vi "Scripting_G1NewToG3New.vi"(0 "VI Refnum":refnum<vi>, 1 "SearchVI":path=path "C:/classes/MainVI/MyGoop2/utils/MyGoop2_New.vi", 2 "GetToModify":path=path "C:/classes/MainVI/MyGoop2/utils/MyGoop2_GetAttributesToModify.vi", 3 "SetToModify":path=path "C:/classes/MainVI/MyGoop2/utils/MyGoop2_SetModifiedAttributes.vi", 5 "error IO":errorcluster) -> (19 "error out":errorcluster)   [LabVIEW 2016]
uses:
  <vilib>/Utility/miscctls.llb/LVPositionTypeDef.ctl
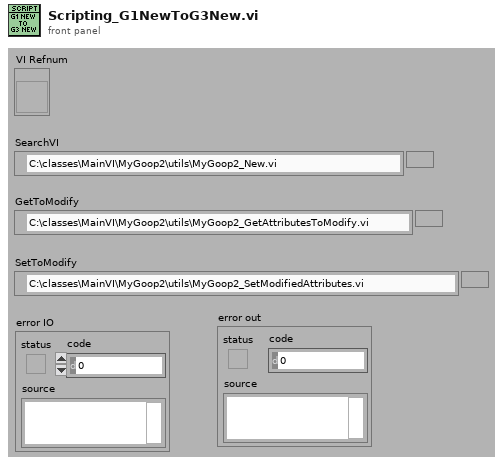
[diagram p1: front panel]
types:
  T1 = cluster{"FoundVI":refnum<vi>, "GetRef":refnum<vi>, "SetRef":refnum<vi>, "Block Diagram":refnum<vi>, "InControl":refnum<vi>, "OutControl":refnum<vi>}
  T2 = typedef "LVPositionTypeDef.ctl" = cluster{"Left":i32, "Top":i32}
  T3 = typedef "LVRectTypeDef.ctl" = cluster{"Left":i16, "Top":i16, "Right":i16, "Bottom":i16}
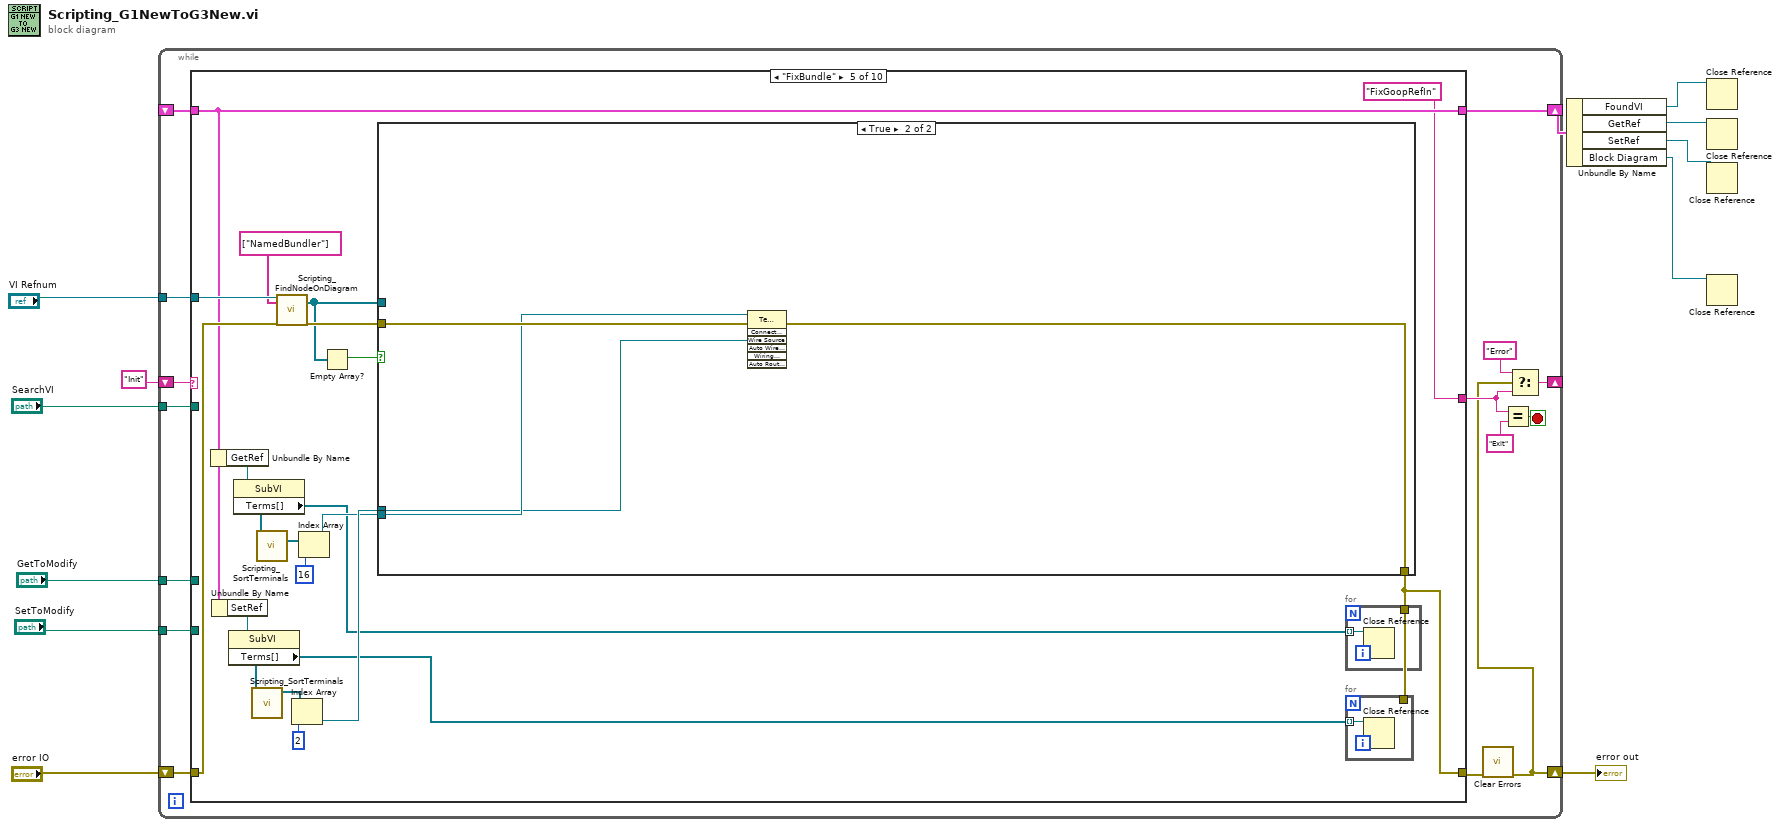
[diagram p0: block diagram]
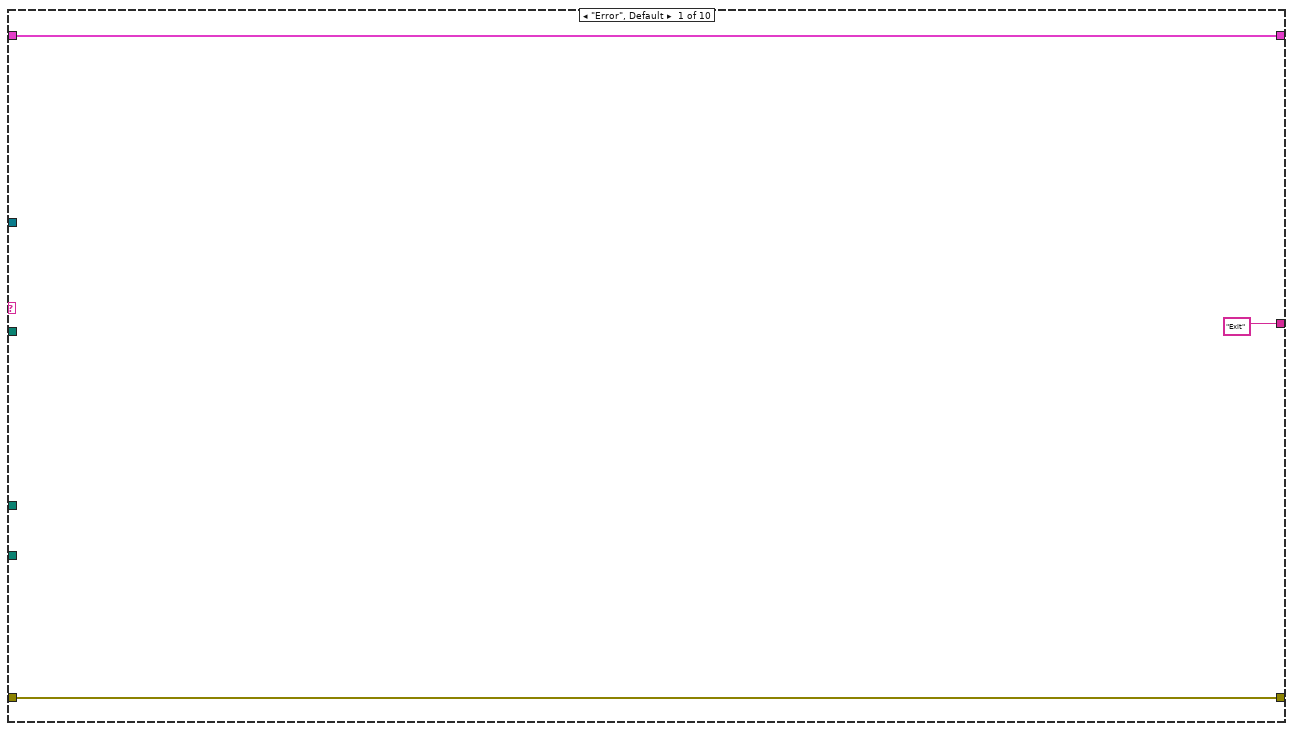
[diagram p2: hidden frame]
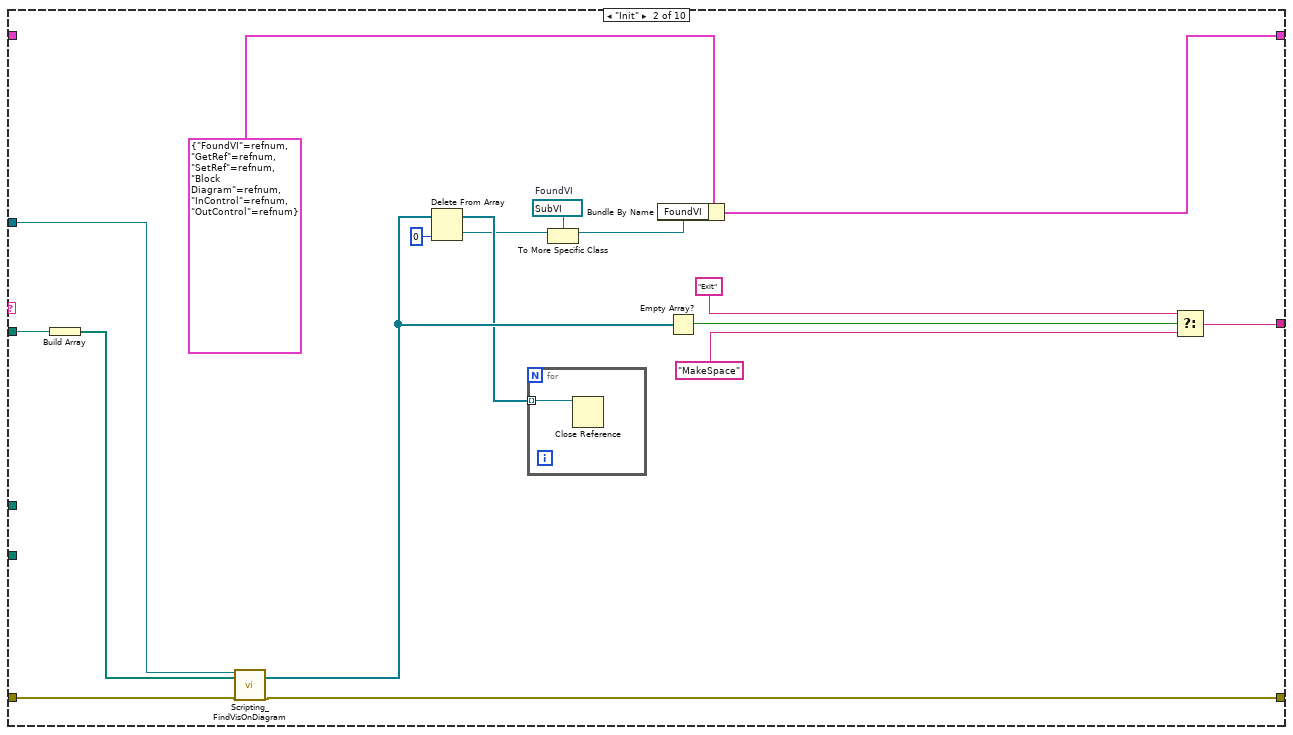
[diagram p3: hidden frame]
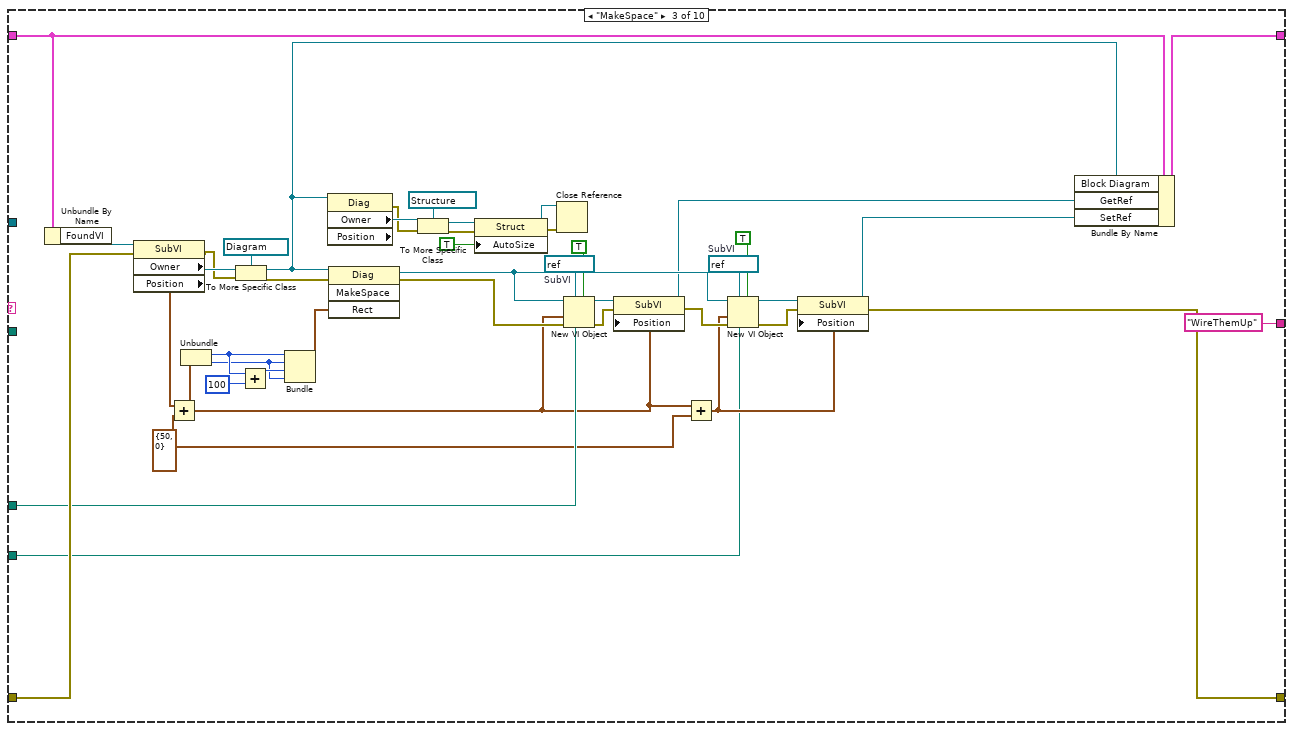
[diagram p4: hidden frame]
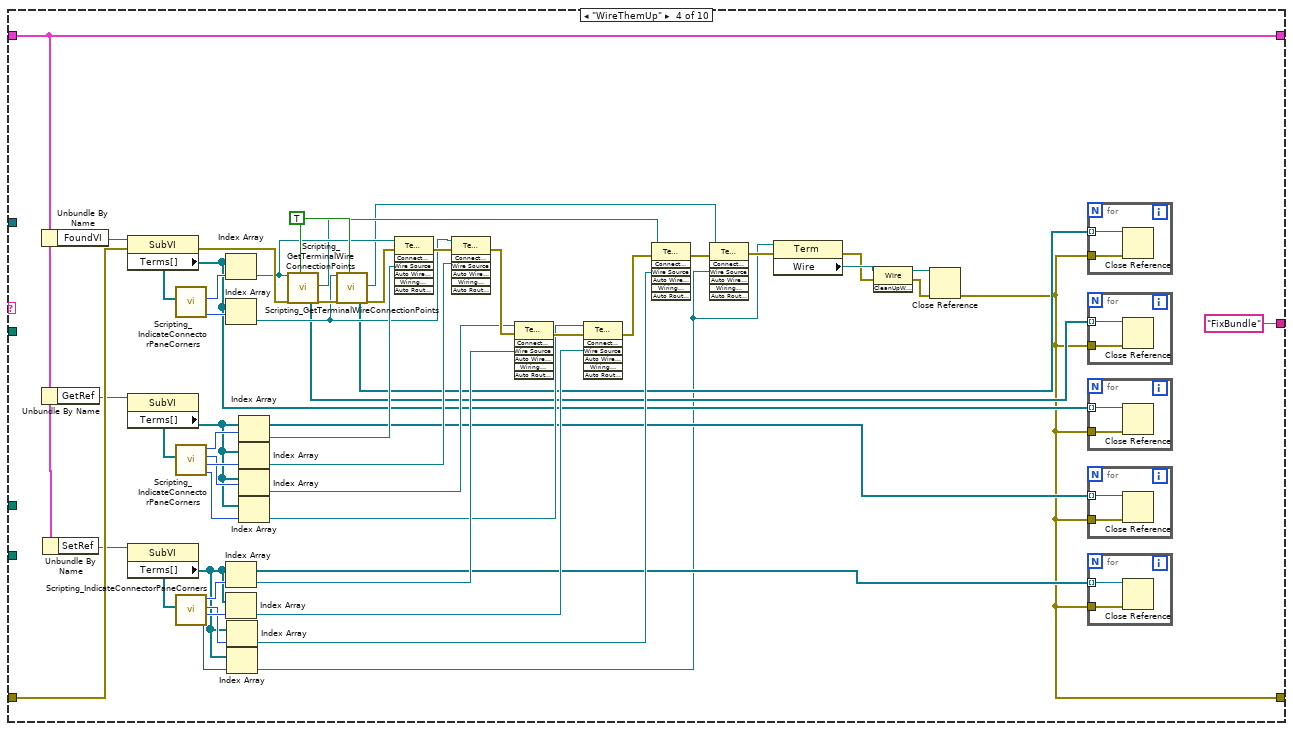
[diagram p5: hidden frame]
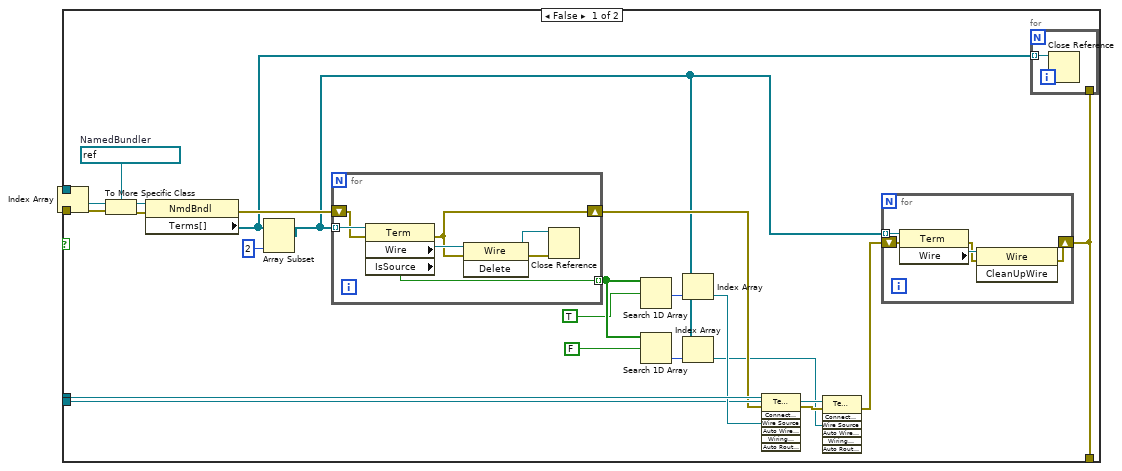
[diagram p6: hidden frame]
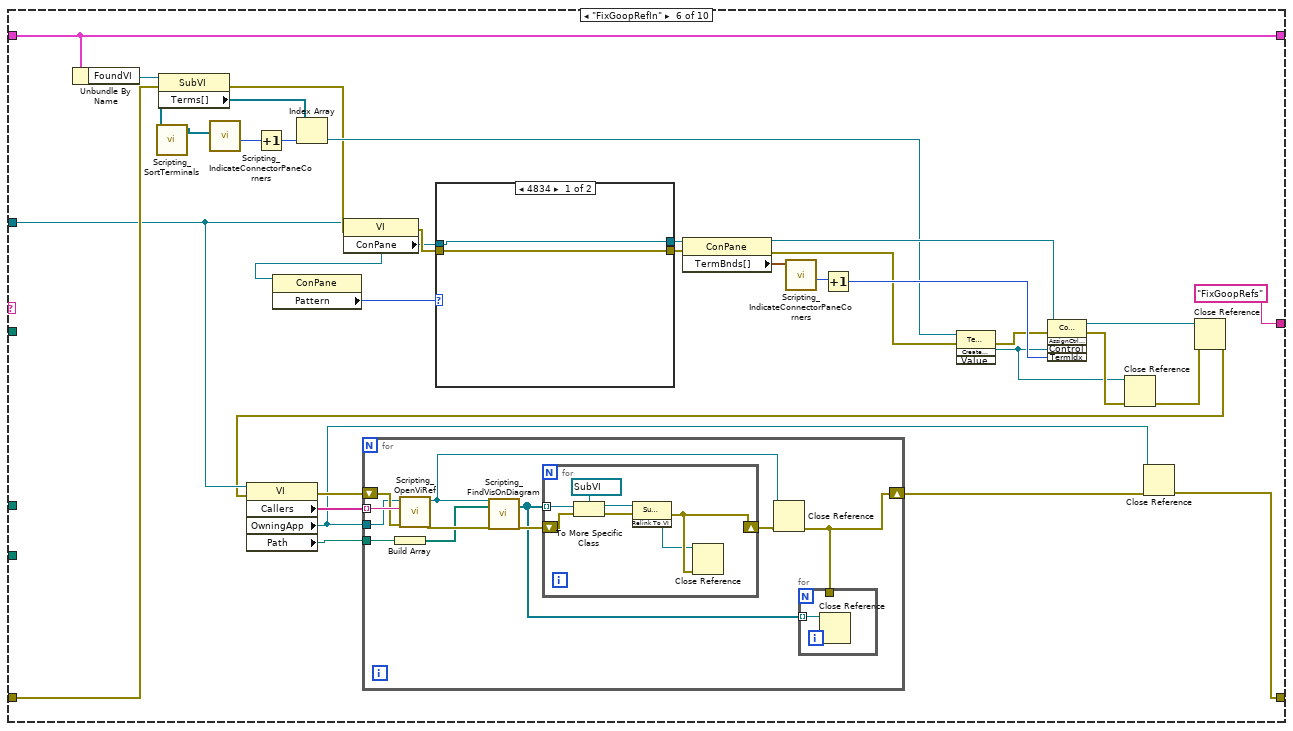
[diagram p7: hidden frame]
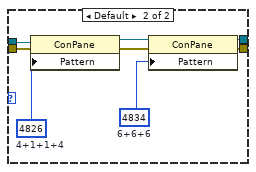
[diagram p8: hidden frame]
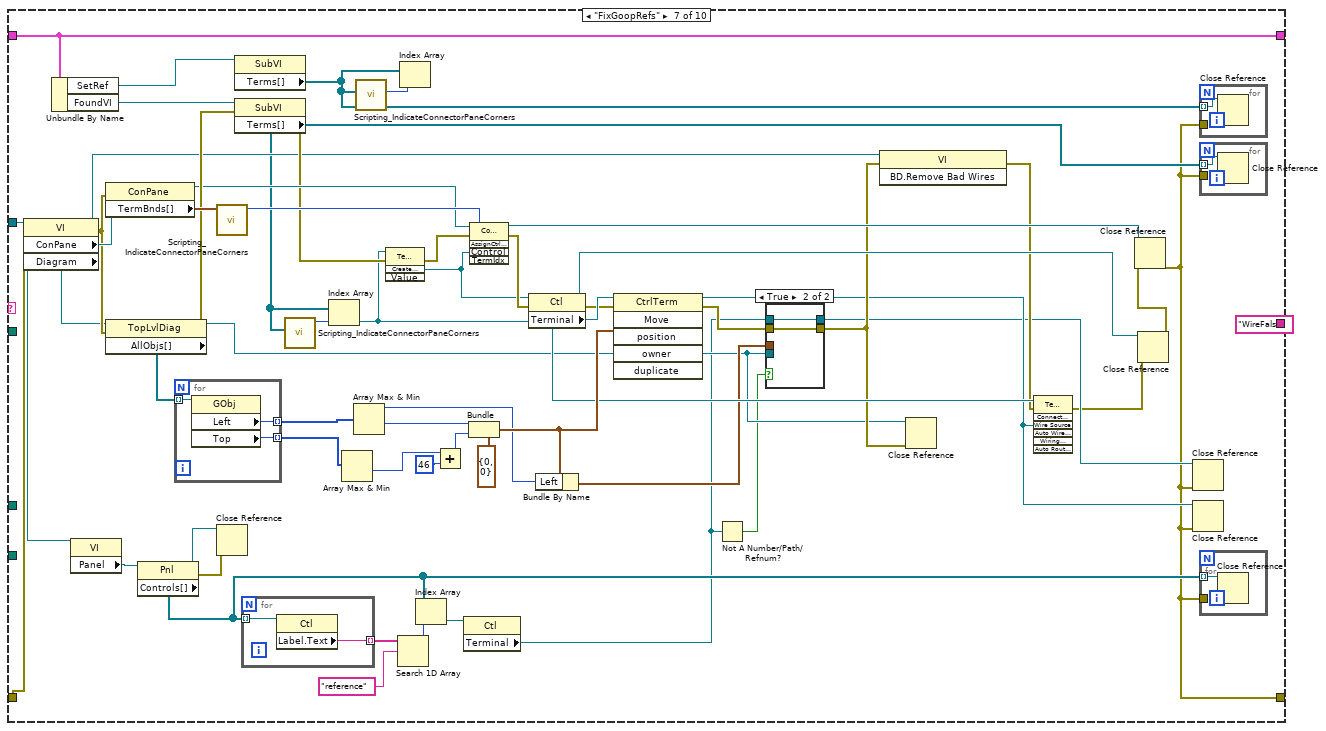
[diagram p9: hidden frame]
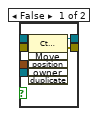
[diagram p10: hidden frame]
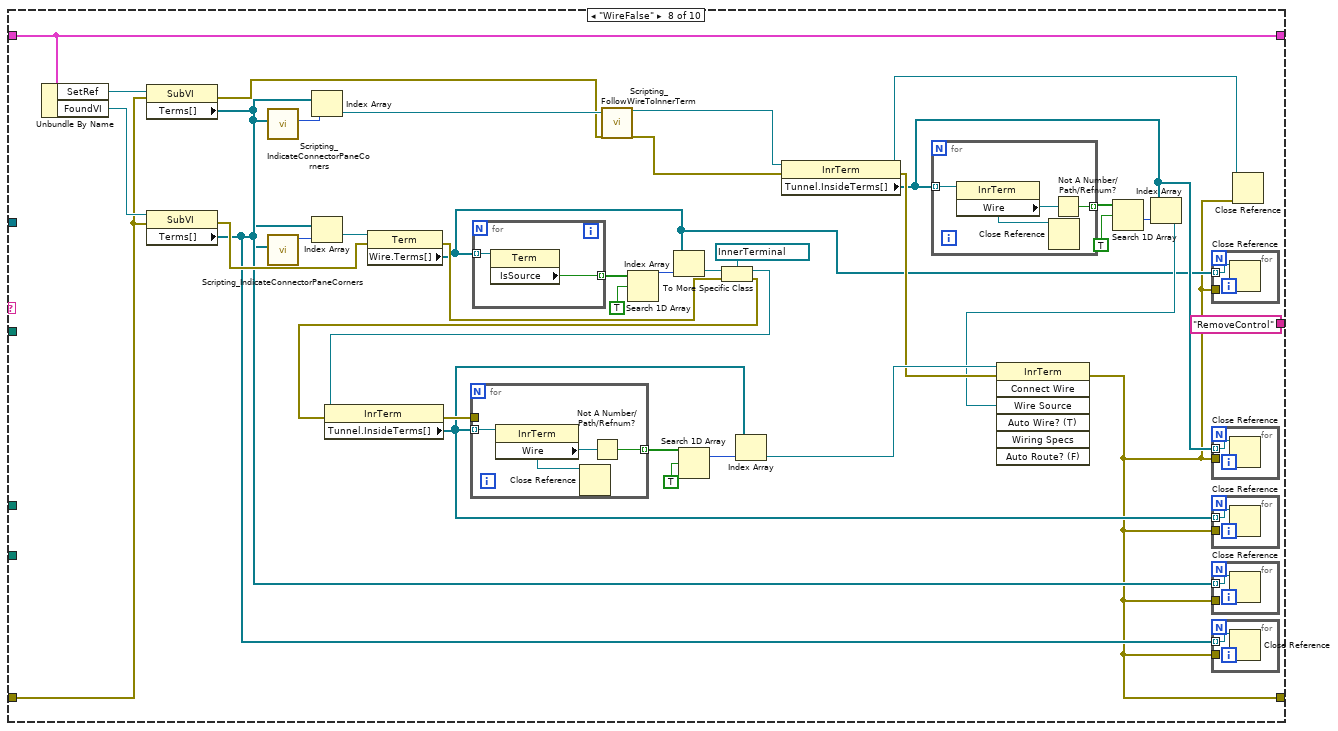
[diagram p11: hidden frame]
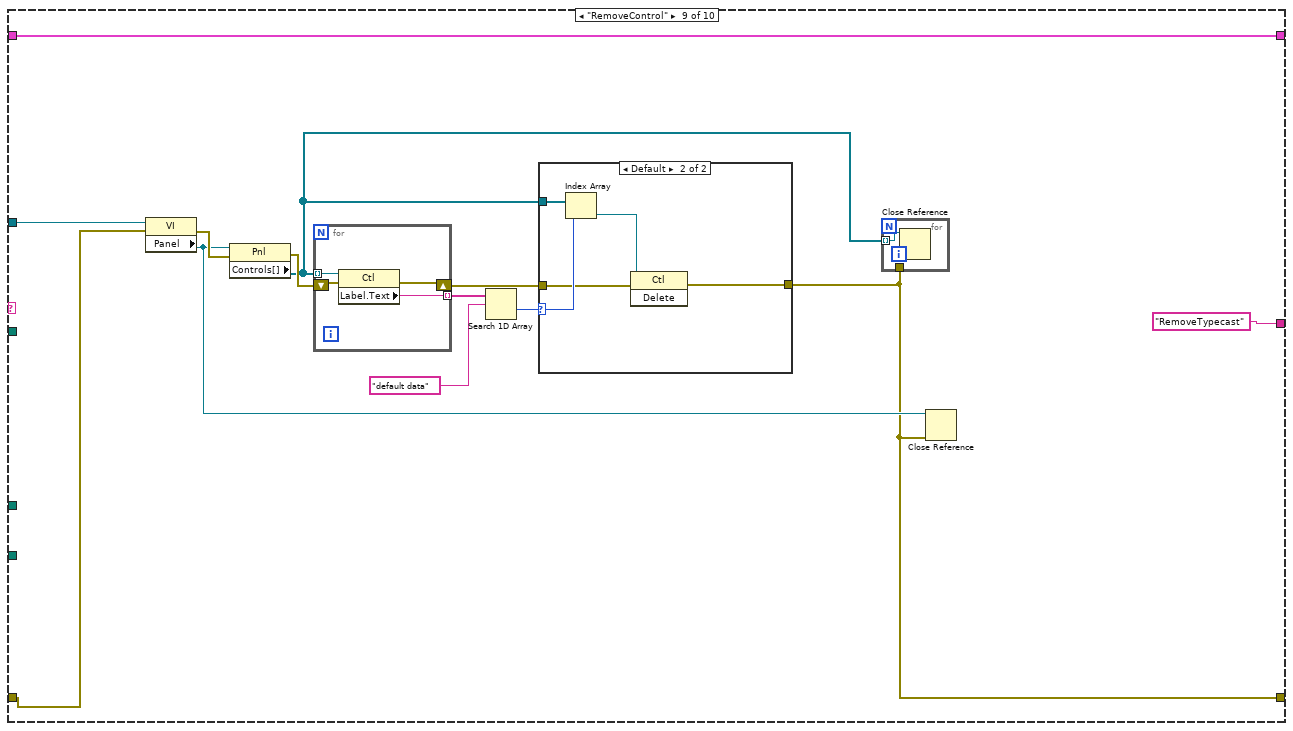
[diagram p12: hidden frame]
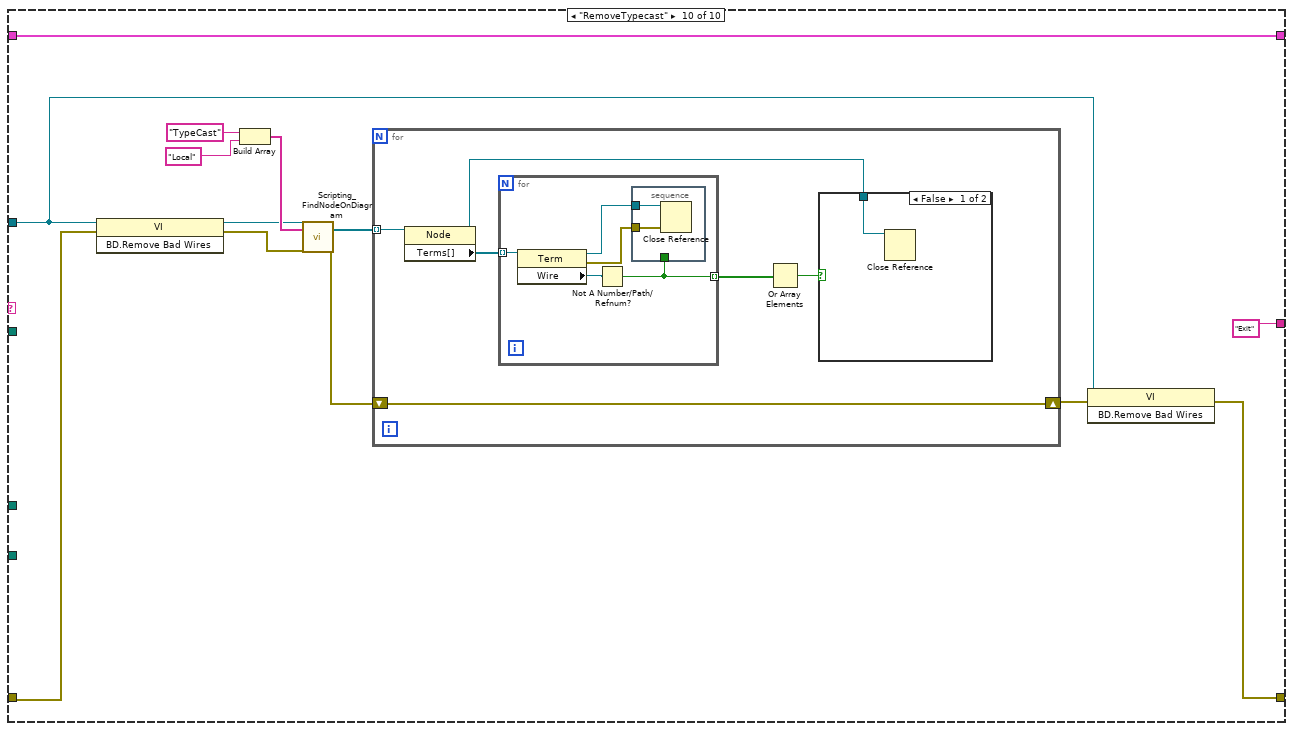
[diagram p14: hidden frame]
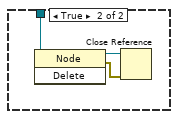
[diagram p15: hidden frame]
diagram:
  n1 = while {
    shift-right: [w13] -> w10
    shift-left: "error IO" -> [w27]
    shift-right: [w25] -> _
    shift-left: "Init" -> [w26]
    shift-right: [w20] -> w6
    shift-left: _ -> [w19]
    tunnel: "VI Refnum" -> [w18]
    tunnel: "SearchVI" -> [w17]
    tunnel: "GetToModify" -> [w16]
    tunnel: "SetToModify" -> [w15]
    stop <- w24 stop-if-true
    n2 = case shown="\"FixBundle\"" w26 {
      tunnel: w27 -> [w28 w45 w90 w138 w166 w226 w319 w357 w401 w429]
      tunnel: [w28 w44 w51 w93 w153 w214 w277 w347 w398 w422] -> w14
      tunnel: ["Exit" w39 "WireThemUp" "FixBundle" "FixGoopRefIn" "FixGoopRefs" "WireFalse" "RemoveControl" "RemoveTypecast" "Exit"] -> w21
      tunnel: [w29 w46 w57 w123 w162 w225 w280 w382 w397 w426] -> w20
      tunnel: w19 -> [w29 _ w58 w123 w162 w225 w280 w382 w397 w426]
      tunnel: w18 -> [_ w43 _ _ w168 w220 w295 _ w402 w424]
      tunnel: w17 -> [_ w36 _ _ _ _ _ _ _ _]
      tunnel: w16 -> [_ _ w83 _ _ _ _ _ _ _]
      tunnel: w15 -> [_ _ w59 _ _ _ _ _ _ _]
      frame "Error", Default {
      }
      frame "Init" {
        w32 = refnum<vi> refnum  # FoundVI
        n3 = Build Array(w36) -> (w35:path[])
        n4 = call <resource>:"Scripting_FindVisOnDiagram.vi"("ViRef"=w43, "VIsToSerachFor/ViName"=w35, "error in (no error)"=w45) -> ("VisFound"=w38:refnum<vi>[], "error out"=w44:errorcluster)  [unwired: 15 in]
        n5 = Delete From Array(array=w38, index=0) -> (deleted portion=w33:refnum<vi>, array with subset deleted=w34:refnum<vi>[])  [unwired: 1 in]
        n6 = for {
          tunnel: w34 -> [w48] mode=indexing
          n7 = Close Reference(reference=w48) -> ()  [unwired: 1 in, 1 out]
        }
        n8 = To More Specific Class(target class=w32, reference=w33) -> (specific class reference=w31:refnum<vi>)  [unwired: 1 in, 1 out]
        n9 = Bundle By Name(cluster=T1 {"FoundVI"=refnum, "GetRef"=refnum, "SetRef"=refnum, "Block Diagram"=refnum, "InControl"=refnum, "OutControl"=refnum}, "FoundVI"=w31) -> (w46:T1)
        n10 = Empty Array?(array=w38) -> (empty?=w42:bool)
        n11 = Select(t="Exit", s=w42, f="MakeSpace") -> (s? t:f=w39:string)
      }
      frame "MakeSpace" {
        w61 = T2 {"Left"=50, "Top"=0} ("y")
        w65 = refnum<vi> refnum  # SubVI
        w86 = refnum<vi> refnum  # SubVI
        n12 = Unbundle By Name(w58) -> ("FoundVI"=w91:refnum<vi>)
        n13 = property class="SubVI"(reference=w91, error in=w90) -> (error out=w87:errorcluster, "Owner"=w88:refnum<vi>, "Position"=w79:T2)  [unwired: 1 out]
        n14 = Add(x=w79, y=w61) -> (x+y=w62:T2)
        n15 = Unbundle(w62) -> ("Left"=w78:i32, "Top"=w75:i32)
        n16 = To More Specific Class(target class=refnum<vi> refnum ("Block Diagram"), reference=w88, error in=w87) -> (specific class reference=w52:refnum<vi>, error out=w72:errorcluster)
        n17 = Add(x=w78, y=i16 100 ("Right")) -> (x+y=w76:i32)
        n18 = Bundle("Left"=w78, "Top"=w75, w76, "Top"=w75) -> (w74:cluster{"Left":i32, "Top":i32, i32, "Top":i32})  [unwired: 1 in]
        n19 = property class="Diag" props=["Owner", "Position"](reference=w52) -> (error out=w49:errorcluster, "Owner"=w71:refnum<vi>)  [unwired: 1 in, 2 out]
        n20 = invoke class="Diag" method="MakeSpace"(reference=w52, error in=w72, "Rect"=w74) -> (reference out=w63:refnum<vi>, error out=w84:errorcluster)  [unwired: 1 in, 2 out]
        n21 = To More Specific Class(target class=refnum<vi> refnum ("Block Diagram"), reference=w71, error in=w49) -> (specific class reference=w70:refnum<vi>, error out=w50:errorcluster)
        n22 = property class="Struct"(reference=w70, error in=w50, "AutoSize"=TRUE ("AutoSize To Fit Contents?")) -> (reference out=w53:refnum<vi>, error out=w54:errorcluster)
        n23 = Close Reference(reference=w53, error in (no error)=w54) -> ()  [unwired: 1 out]
        n24 = New VI Object(vi object class=w86, auto wire? (F)=TRUE, owner refnum=w63, position/next to=w62, 6:w83, 8:w84) -> (object refnum=w82:refnum<vi>, 0:w81:errorcluster)  [unwired: 2 in]
        n25 = property class="SubVI"(reference=w82, error in=w81, "Position"=w62) -> (reference out=w56:refnum<vi>, error out=w64:errorcluster)
        n26 = Add(x=w62, y=w61) -> (x+y=w60:T2)
        n27 = New VI Object(vi object class=w65, auto wire? (F)=TRUE, owner refnum=w63, position/next to=w60, 6:w59, 8:w64) -> (object refnum=w67:refnum<vi>, 0:w68:errorcluster)  [unwired: 2 in]
        n28 = property class="SubVI"(reference=w67, error in=w68, "Position"=w60) -> (reference out=w55:refnum<vi>, error out=w51:errorcluster)
        n29 = Bundle By Name(cluster=w58, "Block Diagram"=w52, "GetRef"=w56, "SetRef"=w55) -> (w57:T1)
      }
      frame "WireThemUp" {
        w134 = TRUE ("RemoveWire(Ture)")
        n30 = Unbundle By Name(w123) -> ("FoundVI"=w139:refnum<vi>)
        n31 = Unbundle By Name(w123) -> ("GetRef"=w133:refnum<vi>)
        n32 = Unbundle By Name(w123) -> ("SetRef"=w124:refnum<vi>)
        n33 = property class="SubVI"(reference=w139, error in=w138) -> (error out=w137:errorcluster, "Terms[]"=w99:refnum<vi>[])  [unwired: 1 out]
        n34 = property class="SubVI"(reference=w133) -> ("Terms[]"=w103:refnum<vi>[])  [unwired: 1 in, 2 out]
        n35 = property class="SubVI"(reference=w124) -> ("Terms[]"=w102:refnum<vi>[])  [unwired: 1 in, 2 out]
        n36 = call <resource>:"Scripting_IndicateConnectorPaneCorners.vi"("Terminals[]"=w99) -> ("RightLower"=w135:i32, "RightTop"=w100:i32)  [unwired: 7 in, 2 out]
        n37 = call <resource>:"Scripting_IndicateConnectorPaneCorners.vi"("Terminals[]"=w103) -> ("RightLower"=w119:i32, "LeftLower"=w131:i32, "RightTop"=w120:i32, "LeftTop"=w132:i32)  [unwired: 7 in]
        n38 = call <resource>:"Scripting_IndicateConnectorPaneCorners.vi"("Terminals[]"=w102) -> ("RightLower"=w111:i32, "LeftLower"=w126:i32, "RightTop"=w112:i32, "LeftTop"=w125:i32)  [unwired: 7 in]
        n39 = Index Array(array=w99, index=w100) -> (element=w113:refnum<vi>)
        n40 = Index Array(array=w99, index=w135) -> (element=w114:refnum<vi>)
        n41 = Index Array(array=w102, index=w125) -> (element=w117:refnum<vi>)
        n42 = Index Array(array=w102, index=w126) -> (element=w116:refnum<vi>)
        n43 = Index Array(array=w102, index=w112) -> (element=w107:refnum<vi>)
        n44 = Index Array(array=w102, index=w111) -> (element=w97:refnum<vi>)
        n45 = Index Array(array=w103, index=w132) -> (element=w129:refnum<vi>)
        n46 = Index Array(array=w103, index=w131) -> (element=w127:refnum<vi>)
        n47 = Index Array(array=w103, index=w120) -> (element=w118:refnum<vi>)
        n48 = Index Array(array=w103, index=w119) -> (element=w115:refnum<vi>)
        n49 = call <resource>:"Scripting_GetTerminalWireConnectionPoints.vi"("Term Refnum In"=w113, "error in"=w137, "RemoveWire(False)"=w134) -> ("AllWireTerminals"=w104:refnum<vi>[], "FirstWireTermDrain"=w110:refnum<vi>, "error out"=w136:errorcluster)  [unwired: 8 in, 6 out]
        n50 = call <resource>:"Scripting_GetTerminalWireConnectionPoints.vi"("Term Refnum In"=w114, "error in"=w136, "RemoveWire(False)"=w134) -> ("AllWireTerminals"=w105:refnum<vi>[], "FirstWireTermDrain"=w109:refnum<vi>, "error out"=w130:errorcluster)  [unwired: 8 in, 6 out]
        n51 = invoke class="Term" method="Connect Wire"(reference=w113, error in=w130, "Wire Source"=w129) -> (error out=w128:errorcluster)  [unwired: 4 in, 6 out]
        n52 = invoke class="Term" method="Connect Wire"(reference=w114, error in=w128, "Wire Source"=w127) -> (error out=w121:errorcluster)  [unwired: 4 in, 6 out]
        n53 = invoke class="Term" method="Connect Wire"(reference=w118, error in=w121, "Wire Source"=w117) -> (error out=w122:errorcluster)  [unwired: 4 in, 6 out]
        n54 = invoke class="Term" method="Connect Wire"(reference=w115, error in=w122, "Wire Source"=w116) -> (error out=w108:errorcluster)  [unwired: 4 in, 6 out]
        n55 = invoke class="Term" method="Connect Wire"(reference=w110, error in=w108, "Wire Source"=w107) -> (error out=w106:errorcluster)  [unwired: 4 in, 6 out]
        n56 = invoke class="Term" method="Connect Wire"(reference=w109, error in=w106, "Wire Source"=w97) -> (error out=w98:errorcluster)  [unwired: 4 in, 6 out]
        n57 = property class="Term"(reference=w97, error in=w98) -> (error out=w95:errorcluster, "Wire"=w96:refnum<vi>)  [unwired: 1 out]
        n58 = invoke class="Wire" method="CleanUpWire"(reference=w96, error in=w95) -> (reference out=w94:refnum<vi>, error out=w92:errorcluster)  [unwired: 1 in, 1 out]
        n59 = Close Reference(reference=w94, error in (no error)=w92) -> (error out=w93:errorcluster)
        n60 = for {
          tunnel: w93 -> [w149]
          tunnel: w105 -> [w148] mode=indexing
          n61 = Close Reference(reference=w148, error in (no error)=w149) -> ()  [unwired: 1 out]
        }
        n62 = for {
          tunnel: w93 -> [w147]
          tunnel: w104 -> [w146] mode=indexing
          n63 = Close Reference(reference=w146, error in (no error)=w147) -> ()  [unwired: 1 out]
        }
        n64 = for {
          tunnel: w93 -> [w145]
          tunnel: w99 -> [w144] mode=indexing
          n65 = Close Reference(reference=w144, error in (no error)=w145) -> ()  [unwired: 1 out]
        }
        n66 = for {
          tunnel: w93 -> [w143]
          tunnel: w103 -> [w142] mode=indexing
          n67 = Close Reference(reference=w142, error in (no error)=w143) -> ()  [unwired: 1 out]
        }
        n68 = for {
          tunnel: w93 -> [w141]
          tunnel: w102 -> [w140] mode=indexing
          n69 = Close Reference(reference=w140, error in (no error)=w141) -> ()  [unwired: 1 out]
        }
      }
      frame "FixBundle" {
        n70 = Unbundle By Name(w162) -> ("GetRef"=w164:refnum<vi>)
        n71 = Unbundle By Name(w162) -> ("SetRef"=w163:refnum<vi>)
        n72 = property class="SubVI"(reference=w163) -> ("Terms[]"=w154:refnum<vi>[])  [unwired: 1 in, 2 out]
        n73 = property class="SubVI"(reference=w164) -> ("Terms[]"=w155:refnum<vi>[])  [unwired: 1 in, 2 out]
        n74 = call <resource>:"Scripting_SortTerminals.vi"("Terminals[]"=w154) -> ("TerminalsOut[]"=w160:refnum<vi>[])  [unwired: 8 in, 2 out]
        n75 = call <resource>:"Scripting_SortTerminals.vi"("Terminals[]"=w155) -> ("TerminalsOut[]"=w157:refnum<vi>[])  [unwired: 8 in, 2 out]
        n76 = call <resource>:"Scripting_FindNodeOnDiagram.vi"("ViRef(Ignored If Not Wired)"=w168, "NodeTypesToSearchFor"=string[] ["NamedBundler"], "error in (no error)"=w166) -> ("Nodes"=w152:refnum<vi>[], "error out"=w165:errorcluster)  [unwired: 15 in]
        n77 = Index Array(array=w160, index=2) -> (element=w159:refnum<vi>)
        n78 = Index Array(array=w157, index=16) -> (element=w156:refnum<vi>)
        n79 = Empty Array?(array=w152) -> (empty?=w150:bool)
        n80 = case shown="True" w150 {
          tunnel: w165 -> [w186 w208]
          tunnel: w159 -> [w181 w206]
          tunnel: w156 -> [w177 w207]
          tunnel: [w170 w205] -> w153
          tunnel: w152 -> [w169 _]
          frame False {
            w190 = refnum<vi> refnum  # NamedBundler
            n81 = Index Array(array=w169) -> (element=w191:refnum<vi>)  [unwired: 1 in]
            n82 = To More Specific Class(target class=w190, reference=w191, error in=w186) -> (specific class reference=w189:refnum<vi>, error out=w187:errorcluster)
            n83 = property class="NmdBndl"(reference=w189, error in=w187) -> (error out=w188:errorcluster, "Terms[]"=w175:refnum<vi>[])  [unwired: 1 out]
            n84 = Array Subset(array=w175, length=2) -> (w172:refnum<vi>[])  [unwired: 1 in]
            n85 = for {
              tunnel: w172 -> [w204] mode=indexing
              shift-right: [w198] -> w176
              shift-left: w188 -> [w201]
              tunnel: [w199] -> w184 mode=indexing
              n86 = property class="Term"(reference=w204, error in=w201) -> (error out=w198:errorcluster, "Wire"=w203:refnum<vi>, "IsSource"=w199:bool)  [unwired: 1 out]
              n87 = invoke class="Wire" method="Delete"(reference=w203, error in=w198) -> (reference out=w202:refnum<vi>, error out=w200:errorcluster)  [unwired: 1 in, 1 out]
              n88 = Close Reference(reference=w202, error in (no error)=w200) -> ()  [unwired: 1 out]
            }
            n89 = Search 1D Array(1D array=w184, element=TRUE) -> (index of element=w180:i32)  [unwired: 1 in]
            n90 = Search 1D Array(1D array=w184, element=FALSE) -> (index of element=w174:i32)  [unwired: 1 in]
            n91 = Index Array(array=w172, index=w180) -> (element=w179:refnum<vi>)
            n92 = Index Array(array=w172, index=w174) -> (element=w173:refnum<vi>)
            n93 = invoke class="Term" method="Connect Wire"(reference=w181, error in=w176, "Wire Source"=w179) -> (error out=w178:errorcluster)  [unwired: 4 in, 6 out]
            n94 = invoke class="Term" method="Connect Wire"(reference=w177, error in=w178, "Wire Source"=w173) -> (error out=w171:errorcluster)  [unwired: 4 in, 6 out]
            n95 = for {
              tunnel: w172 -> [w196] mode=indexing
              shift-right: [w192] -> w170
              shift-left: w171 -> [w194]
              n96 = property class="Term"(reference=w196, error in=w194) -> (error out=w193:errorcluster, "Wire"=w195:refnum<vi>)  [unwired: 1 out]
              n97 = invoke class="Wire" method="CleanUpWire"(reference=w195, error in=w193) -> (error out=w192:errorcluster)  [unwired: 1 in, 2 out]
            }
            n98 = for {
              tunnel: w175 -> [w197] mode=indexing
              tunnel: w170 -> [_]
              n99 = Close Reference(reference=w197) -> ()  [unwired: 1 in, 1 out]
            }
          }
          frame True {
            n100 = invoke class="Term" method="Connect Wire"(reference=w207, error in=w208, "Wire Source"=w206) -> (error out=w205:errorcluster)  [unwired: 4 in, 6 out]
          }
        }
        n101 = for {
          tunnel: w155 -> [w210] mode=indexing
          tunnel: w153 -> [_]
          n102 = Close Reference(reference=w210) -> ()  [unwired: 1 in, 1 out]
        }
        n103 = for {
          tunnel: w154 -> [w209] mode=indexing
          tunnel: w153 -> [_]
          n104 = Close Reference(reference=w209) -> ()  [unwired: 1 in, 1 out]
        }
      }
      frame "FixGoopRefIn" {
        n105 = Unbundle By Name(w225) -> ("FoundVI"=w239:refnum<vi>)
        n106 = property class="SubVI"(reference=w239, error in=w226) -> (error out=w227:errorcluster, "Terms[]"=w237:refnum<vi>[])  [unwired: 1 out]
        n107 = call <resource>:"Scripting_SortTerminals.vi"("Terminals[]"=w237) -> ("TerminalsOut[]"=w236:refnum<vi>[])  [unwired: 8 in, 2 out]
        n108 = call <resource>:"Scripting_IndicateConnectorPaneCorners.vi"("Terminals[]"=w236) -> ("LeftLower"=w238:i32)  [unwired: 7 in, 3 out]
        n109 = Increment(x=w238) -> (x+1=w243:i32)
        n110 = Index Array(array=w237, index=w243) -> (element=w229:refnum<vi>)
        n111 = property class="VI"(reference=w220, error in=w227) -> (error out=w223:errorcluster, "ConPane"=w212:refnum<vi>)  [unwired: 1 out]
        n112 = property class="ConPane"(reference=w212) -> ("Pattern"=w211:u32)  [unwired: 1 in, 2 out]
        n113 = case shown="4834" w211 {
          tunnel: w212 -> [w245 w253]
          tunnel: w223 -> [w244 w252]
          tunnel: [w244 w247] -> w222
          tunnel: [w245 w246] -> w221
          frame 4834 {
          }
          frame Default {
            w251 = u32 4826  # 4+1+1+4
            w248 = u32 4834  # 6+6+6
            n114 = property class="ConPane"(reference=w253, error in=w252, "Pattern"=w251) -> (reference out=w250:refnum<vi>, error out=w249:errorcluster)
            n115 = property class="ConPane"(reference=w250, error in=w249, "Pattern"=w248) -> (reference out=w246:refnum<vi>, error out=w247:errorcluster)
          }
        }
        n116 = property class="ConPane"(reference=w221, error in=w222) -> (reference out=w235:refnum<vi>, error out=w228:errorcluster, "TermBnds[]"=w241:T3[])
        n117 = call <resource>:"Scripting_IndicateConnectorPaneCorners.vi"("TermBnds[]"=w241) -> ("LeftLower"=w240:i32)  [unwired: 7 in, 3 out]
        n118 = Increment(x=w240) -> (x+1=w234:i32)
        n119 = invoke class="Term" method="Create Control"(reference=w229, error in=w228) -> (error out=w233:errorcluster, "Create Control"=w232:refnum<vi>)  [unwired: 2 in, 2 out]
        n120 = invoke class="ConPane" method="AssignCtrlToTerm"(reference=w235, error in=w233, "Control"=w232, "TermIdx"=w234) -> (reference out=w230:refnum<vi>, error out=w242:errorcluster)  [unwired: 1 in, 3 out]
        n121 = Close Reference(reference=w232, error in (no error)=w242) -> (error out=w231:errorcluster)
        n122 = Close Reference(reference=w230, error in (no error)=w231) -> (error out=w216:errorcluster)
        n123 = property class="VI"(reference=w220, error in=w216) -> (error out=w218:errorcluster, "Callers"=w219:string[], "OwningApp"=w213:refnum<vi>, "Path"=w217:path)  [unwired: 1 out]
        n124 = for {
          tunnel: w219 -> [w264] mode=indexing
          tunnel: w217 -> [w261]
          tunnel: w213 -> [w257]
          shift-right: [w254] -> w215
          shift-left: w218 -> [w263]
          n125 = Build Array(w261) -> (w260:path[])
          n126 = call <resource>:"Scripting_OpenViRef.vi"("error in"=w263, "ViPath/ViName/Viref"=w264, "AppRef"=w257) -> ("error out"=w262:errorcluster, "vi reference"=w255:refnum<vi>)  [unwired: 6 in, 1 out]
          n127 = call <resource>:"Scripting_FindVisOnDiagram.vi"("ViRef"=w255, "VIsToSerachFor/ViName"=w260, "error in (no error)"=w262) -> ("VisFound"=w258:refnum<vi>[], "error out"=w259:errorcluster)  [unwired: 15 in]
          n128 = for {
            tunnel: w258 -> [w271] mode=indexing
            shift-right: [w267] -> w256
            shift-left: w259 -> [w270]
            n129 = To More Specific Class(target class=refnum<vi> refnum ("WhileLoop"), reference=w271, error in=w270) -> (specific class reference=w269:refnum<vi>, error out=w268:errorcluster)
            n130 = invoke class="SubVI" method="Relink To VI"(reference=w269, error in=w268) -> (error out=w267:errorcluster, "Relink To VI"=w266:refnum<vi>)  [unwired: 1 in, 1 out]
            n131 = Close Reference(reference=w266, error in (no error)=w267) -> ()  [unwired: 1 out]
          }
          n132 = Close Reference(reference=w255, error in (no error)=w256) -> (error out=w254:errorcluster)
          n133 = for {
            tunnel: w258 -> [w265] mode=indexing
            tunnel: w254 -> [_]
            n134 = Close Reference(reference=w265) -> ()  [unwired: 1 in, 1 out]
          }
        }
        n135 = Close Reference(reference=w213, error in (no error)=w215) -> (error out=w214:errorcluster)
      }
      frame "FixGoopRefs" {
        n136 = property class="VI"(reference=w295, error in=w319) -> (reference out=w299:refnum<vi>, error out=w304:errorcluster, "ConPane"=w328:refnum<vi>, "Diagram"=w303:refnum<vi>)
        n137 = Unbundle By Name(w280) -> ("SetRef"=w289:refnum<vi>, "FoundVI"=w309:refnum<vi>)
        n138 = property class="VI"(reference=w295) -> ("Panel"=w294:refnum<vi>)  [unwired: 1 in, 2 out]
        n139 = property class="ConPane"(reference=w328, error in=w304) -> (reference out=w318:refnum<vi>, "TermBnds[]"=w327:T3[])  [unwired: 1 out]
        n140 = property class="TopLvlDiag"(reference=w303, error in=w304) -> (reference out=w283:refnum<vi>, error out=w323:errorcluster, "AllObjs[]"=w314:refnum<vi>[])
        n141 = property class="Pnl"(reference=w294) -> (reference out=w285:refnum<vi>, error out=w286:errorcluster, "Controls[]"=w287:refnum<vi>[])  [unwired: 1 in]
        n142 = for {
          tunnel: w314 -> [w345] mode=indexing
          tunnel: [w344] -> w326 mode=indexing
          tunnel: [w343] -> w325 mode=indexing
          n143 = property class="GObj"(reference=w345) -> ("Left"=w344:i32, "Top"=w343:i32)  [unwired: 1 in, 2 out]
        }
        n144 = call <resource>:"Scripting_IndicateConnectorPaneCorners.vi"("TermBnds[]"=w327) -> ("LeftTop"=w321:i32)  [unwired: 7 in, 3 out]
        n145 = Close Reference(reference=w285, error in (no error)=w286) -> ()  [unwired: 1 out]
        n146 = property class="SubVI"(reference=w289) -> ("Terms[]"=w281:refnum<vi>[])  [unwired: 1 in, 2 out]
        n147 = property class="SubVI"(reference=w309, error in=w323) -> (error out=w310:errorcluster, "Terms[]"=w282:refnum<vi>[])  [unwired: 1 out]
        n148 = for {
          tunnel: [w342] -> w298 mode=indexing
          tunnel: w287 -> [w341] mode=indexing
          n149 = property class="Ctl"(reference=w341) -> ("Label.Text"=w342:string)  [unwired: 1 in, 2 out]
        }
        n150 = call <resource>:"Scripting_IndicateConnectorPaneCorners.vi"("Terminals[]"=w282) -> ("LeftTop"=w329:i32)  [unwired: 7 in, 3 out]
        n151 = Index Array(array=w282, index=w329) -> (element=w301:refnum<vi>)
        n152 = Array Max & Min(array=w325) -> (min value=w306:i32)  [unwired: 3 out]
        n153 = Array Max & Min(array=w326) -> (max value=w290:i32, min value=w307:i32)  [unwired: 2 out]
        n154 = call <resource>:"Scripting_IndicateConnectorPaneCorners.vi"("Terminals[]"=w281) -> ("RightTop"=w288:i32)  [unwired: 7 in, 3 out]
        n155 = invoke class="Term" method="Create Control"(reference=w301, error in=w310) -> (error out=w311:errorcluster, "Create Control"=w312:refnum<vi>)  [unwired: 2 in, 2 out]
        n156 = Search 1D Array(1D array=w298, element="reference") -> (index of element=w297:i32)  [unwired: 1 in]
        n157 = Index Array(array=w281, index=w288) -> ()  [unwired: 1 out]
        n158 = Index Array(array=w287, index=w297) -> (element=w296:refnum<vi>)
        n159 = Add(x=w306, y=u32 46) -> (x+y=w305:u32)
        n160 = property class="Ctl"(reference=w296) -> ("Terminal"=w274:refnum<vi>)  [unwired: 1 in, 2 out]
        n161 = Bundle(cluster=T2 {"Left"=0, "Top"=0} ("position"), "Left"=w307, "Top"=w305) -> (w302:T2)
        n162 = invoke class="ConPane" method="AssignCtrlToTerm"(reference=w318, error in=w311, "Control"=w312, "TermIdx"=w321) -> (reference out=w324:refnum<vi>, error out=w317:errorcluster)  [unwired: 1 in, 3 out]
        n163 = property class="Ctl"(reference=w312, error in=w317) -> (reference out=w315:refnum<vi>, error out=w313:errorcluster, "Terminal"=w316:refnum<vi>)
        n164 = Bundle By Name(cluster=w302, "Left"=w290) -> (w291:T2)
        n165 = invoke class="CtrlTerm" method="Move"(reference=w316, error in=w313, "position"=w302, "owner"=w283) -> (reference out=w279:refnum<vi>, error out=w292:errorcluster)  [unwired: 2 in, 4 out]
        n166 = Not A Number/Path/Refnum?(number/path/refnum=w274) -> (NaN/Path/Refnum?=w273:bool)
        n167 = case shown="True" w273 {
          tunnel: w292 -> [w335 w336]
          tunnel: w291 -> [w334 _]
          tunnel: [w333 w336] -> w284
          tunnel: w283 -> [w332 _]
          tunnel: [w331 w337] -> w278
          tunnel: w274 -> [w330 w337]
          frame False {
            n168 = invoke class="CtrlTerm" method="Move"(reference=w330, error in=w335, "position"=w334, "owner"=w332) -> (reference out=w331:refnum<vi>, error out=w333:errorcluster)  [unwired: 2 in, 4 out]
          }
          frame True {
          }
        }
        n169 = invoke class="VI" method="BD.Remove Bad Wires"(reference=w299, error in=w284) -> (error out=w300:errorcluster)  [unwired: 1 in, 2 out]
        n170 = Close Reference(reference=w283, error in (no error)=w284) -> ()  [unwired: 1 out]
        n171 = invoke class="Term" method="Connect Wire"(reference=w301, error in=w300, "Wire Source"=w279) -> (error out=w276:errorcluster)  [unwired: 4 in, 6 out]
        n172 = Close Reference(reference=w315, error in (no error)=w276) -> (error out=w275:errorcluster)
        n173 = Close Reference(reference=w324, error in (no error)=w275) -> (error out=w277:errorcluster)
        n174 = Close Reference(reference=w278, error in (no error)=w277) -> ()  [unwired: 1 out]
        n175 = Close Reference(reference=w279, error in (no error)=w277) -> ()  [unwired: 1 out]
        n176 = for {
          tunnel: w281 -> [w338] mode=indexing
          tunnel: w277 -> [_]
          n177 = Close Reference(reference=w338) -> ()  [unwired: 1 in, 1 out]
        }
        n178 = for {
          tunnel: w282 -> [w339] mode=indexing
          tunnel: w277 -> [_]
          n179 = Close Reference(reference=w339) -> ()  [unwired: 1 in, 1 out]
        }
        n180 = for {
          tunnel: w287 -> [w340] mode=indexing
          tunnel: w277 -> [_]
          n181 = Close Reference(reference=w340) -> ()  [unwired: 1 in, 1 out]
        }
      }
      frame "WireFalse" {
        n182 = Unbundle By Name(w382) -> ("SetRef"=w380:refnum<vi>, "FoundVI"=w371:refnum<vi>)
        n183 = property class="SubVI"(reference=w380, error in=w357) -> (error out=w349:errorcluster, "Terms[]"=w352:refnum<vi>[])  [unwired: 1 out]
        n184 = property class="SubVI"(reference=w371, error in=w357) -> (error out=w360:errorcluster, "Terms[]"=w351:refnum<vi>[])  [unwired: 1 out]
        n185 = call <resource>:"Scripting_IndicateConnectorPaneCorners.vi"("Terminals[]"=w352) -> ("RightTop"=w381:i32)  [unwired: 7 in, 3 out]
        n186 = call <resource>:"Scripting_IndicateConnectorPaneCorners.vi"("Terminals[]"=w351) -> ("LeftTop"=w370:i32)  [unwired: 7 in, 3 out]
        n187 = Index Array(array=w352, index=w381) -> (element=w379:refnum<vi>)
        n188 = Index Array(array=w351, index=w370) -> (element=w374:refnum<vi>)
        n189 = property class="Term"(reference=w374, error in=w360) -> (error out=w359:errorcluster, "Wire.Terms[]"=w353:refnum<vi>[])  [unwired: 1 out]
        n190 = for {
          tunnel: w353 -> [w393] mode=indexing
          tunnel: [w392] -> w373 mode=indexing
          n191 = property class="Term"(reference=w393) -> ("IsSource"=w392:bool)  [unwired: 1 in, 2 out]
        }
        n192 = call <resource>:"Scripting_FollowWireToInnerTerm.vi"("Term Refnum"=w379, "error in"=w349) -> ("reference"=w378:refnum<vi>, "error out"=w348:errorcluster)  [unwired: 16 in]
        n193 = Search 1D Array(1D array=w373, element=TRUE) -> (index of element=w369:i32)  [unwired: 1 in]
        n194 = Index Array(array=w353, index=w369) -> (element=w367:refnum<vi>)
        n195 = To More Specific Class(target class=refnum<vi> refnum ("reference"), reference=w367, error in=w359) -> (specific class reference=w366:refnum<vi>, error out=w350:errorcluster)
        n196 = property class="InrTerm"(reference=w366, error in=w350) -> (error out=w361:errorcluster, "Tunnel.InsideTerms[]"=w355:refnum<vi>[])  [unwired: 1 out]
        n197 = for {
          tunnel: w355 -> [w391] mode=indexing
          tunnel: [w390] -> w363 mode=indexing
          tunnel: w361 -> [_]
          n198 = property class="InrTerm"(reference=w391) -> ("Wire"=w389:refnum<vi>)  [unwired: 1 in, 2 out]
          n199 = Close Reference(reference=w389) -> ()  [unwired: 1 in, 1 out]
          n200 = Not A Number/Path/Refnum?(number/path/refnum=w389) -> (NaN/Path/Refnum?=w390:bool)
        }
        n201 = Search 1D Array(1D array=w363, element=TRUE) -> (index of element=w364:i32)  [unwired: 1 in]
        n202 = Index Array(array=w355, index=w364) -> (element=w362:refnum<vi>)
        n203 = property class="InrTerm"(reference=w378, error in=w348) -> (reference out=w346:refnum<vi>, error out=w358:errorcluster, "Tunnel.InsideTerms[]"=w356:refnum<vi>[])
        n204 = for {
          tunnel: w356 -> [w396] mode=indexing
          tunnel: [w395] -> w375 mode=indexing
          n205 = property class="InrTerm"(reference=w396) -> ("Wire"=w394:refnum<vi>)  [unwired: 1 in, 2 out]
          n206 = Close Reference(reference=w394) -> ()  [unwired: 1 in, 1 out]
          n207 = Not A Number/Path/Refnum?(number/path/refnum=w394) -> (NaN/Path/Refnum?=w395:bool)
        }
        n208 = Search 1D Array(1D array=w375, element=TRUE) -> (index of element=w377:i32)  [unwired: 1 in]
        n209 = Index Array(array=w356, index=w377) -> (element=w354:refnum<vi>)
        n210 = invoke class="InrTerm" method="Connect Wire"(reference=w362, error in=w358, "Wire Source"=w354) -> (error out=w347:errorcluster)  [unwired: 4 in, 6 out]
        n211 = for {
          tunnel: w353 -> [w386] mode=indexing
          tunnel: w347 -> [_]
          n212 = Close Reference(reference=w386) -> ()  [unwired: 1 in, 1 out]
        }
        n213 = for {
          tunnel: w356 -> [w388] mode=indexing
          tunnel: w347 -> [_]
          n214 = Close Reference(reference=w388) -> ()  [unwired: 1 in, 1 out]
        }
        n215 = for {
          tunnel: w355 -> [w387] mode=indexing
          tunnel: w347 -> [_]
          n216 = Close Reference(reference=w387) -> ()  [unwired: 1 in, 1 out]
        }
        n217 = for {
          tunnel: w352 -> [w385] mode=indexing
          tunnel: w347 -> [_]
          n218 = Close Reference(reference=w385) -> ()  [unwired: 1 in, 1 out]
        }
        n219 = for {
          tunnel: w351 -> [w384] mode=indexing
          tunnel: w347 -> [_]
          n220 = Close Reference(reference=w384) -> ()  [unwired: 1 in, 1 out]
        }
        n221 = Close Reference(reference=w346, error in (no error)=w347) -> ()  [unwired: 1 out]
      }
      frame "RemoveControl" {
        n222 = property class="VI"(reference=w402, error in=w401) -> (error out=w406:errorcluster, "Panel"=w399:refnum<vi>)  [unwired: 1 out]
        n223 = property class="Pnl"(reference=w399, error in=w406) -> (error out=w404:errorcluster, "Controls[]"=w400:refnum<vi>[])  [unwired: 1 out]
        n224 = for {
          tunnel: w400 -> [w420] mode=indexing
          tunnel: [w419] -> w408 mode=indexing
          shift-right: [w417] -> w403
          shift-left: w404 -> [w418]
          n225 = property class="Ctl"(reference=w420, error in=w418) -> (error out=w417:errorcluster, "Label.Text"=w419:string)  [unwired: 1 out]
        }
        n226 = Search 1D Array(1D array=w408, element="default data") -> (index of element=w405:i32)  [unwired: 1 in]
        n227 = case shown="Default" w405 {
          selector: w405 -> [_ w415]
          tunnel: w400 -> [_ w416]
          tunnel: w403 -> [w411 w413]
          tunnel: [w411 w412] -> w398
          frame -1 {
          }
          frame Default {
            n228 = Index Array(array=w416, index=w415) -> (element=w414:refnum<vi>)
            n229 = invoke class="Ctl" method="Delete"(reference=w414, error in=w413) -> (error out=w412:errorcluster)  [unwired: 1 in, 2 out]
          }
        }
        n230 = for {
          tunnel: w400 -> [w410] mode=indexing
          tunnel: w398 -> [_]
          n231 = Close Reference(reference=w410) -> ()  [unwired: 1 in, 1 out]
        }
        n232 = Close Reference(reference=w399, error in (no error)=w398) -> ()  [unwired: 1 out]
      }
      frame "RemoveTypecast" {
        n233 = invoke class="VI" method="BD.Remove Bad Wires"(reference=w424, error in=w429) -> (reference out=w430:refnum<vi>, error out=w428:errorcluster)  [unwired: 1 in, 1 out]
        n234 = Build Array("TypeCast", "Local") -> (w431:string[])
        n235 = call <resource>:"Scripting_FindNodeOnDiagram.vi"("ViRef(Ignored If Not Wired)"=w430, "NodeTypesToSearchFor"=w431, "error in (no error)"=w428) -> ("Nodes"=w427:refnum<vi>[], "error out"=w423:errorcluster)  [unwired: 15 in]
        n236 = for {
          tunnel: w427 -> [w439] mode=indexing
          shift-right: [w434] -> w425
          shift-left: w423 -> [w434]
          n237 = property class="Node"(reference=w439) -> (reference out=w436:refnum<vi>, "Terms[]"=w438:refnum<vi>[])  [unwired: 1 in, 1 out]
          n238 = for {
            tunnel: w438 -> [w448] mode=indexing
            tunnel: [w445] -> w437 mode=indexing
            n239 = property class="Term"(reference=w448) -> (reference out=w444:refnum<vi>, error out=w446:errorcluster, "Wire"=w447:refnum<vi>)  [unwired: 1 in]
            n240 = Not A Number/Path/Refnum?(number/path/refnum=w447) -> (NaN/Path/Refnum?=w445:bool)
            n241 = stacked-sequence {
              tunnel: w446 -> [w450]
              tunnel: w445 -> [_]
              tunnel: w444 -> [w449]
              frame #0 {
                n242 = Close Reference(reference=w449, error in (no error)=w450) -> ()  [unwired: 1 out]
              }
            }
          }
          n243 = Or Array Elements(Boolean array=w437) -> (logical OR=w435:bool)
          n244 = case shown="False" w435 {
            tunnel: w436 -> [w440 w443]
            frame False {
              n245 = Close Reference(reference=w440) -> ()  [unwired: 1 in, 1 out]
            }
            frame True {
              n246 = invoke class="Node" method="Delete"(reference=w443) -> (reference out=w442:refnum<vi>, error out=w441:errorcluster)  [unwired: 2 in, 1 out]
              n247 = Close Reference(reference=w442, error in (no error)=w441) -> ()  [unwired: 1 out]
            }
          }
        }
        n248 = invoke class="VI" method="BD.Remove Bad Wires"(reference=w424, error in=w425) -> (error out=w422:errorcluster)  [unwired: 1 in, 2 out]
      }
    }
    n249 = call <vilib>:"Clear Errors.vi"("error in (no error)"=w14) -> ("error out"=w13:errorcluster)  [unwired: 5 in, 1 out]
    n250 = Equal?(x=w21, y="Exit") -> (x = y?=w24:bool)
    n251 = Select(t="Error", s=w13, f=w21) -> (s? t:f=w25:string)
  }
  "error out" <- w10
  n252 = Unbundle By Name(w6) -> ("FoundVI"=w5:refnum<vi>, "GetRef"=w4:refnum<vi>, "SetRef"=w3:refnum<vi>, "Block Diagram"=w2:refnum<vi>)
  n253 = Close Reference(reference=w5) -> ()  [unwired: 1 in, 1 out]
  n254 = Close Reference(reference=w4) -> ()  [unwired: 1 in, 1 out]
  n255 = Close Reference(reference=w3) -> ()  [unwired: 1 in, 1 out]
  n256 = Close Reference(reference=w2) -> ()  [unwired: 1 in, 1 out]
